vi "Splite Single-line Message.vi"(2 "Single-line Text":string) -> (6 "Operator":string, 7 "State":string, 9 "Args":string, 10 "Source/target":string)   [LabVIEW 2017, in "Communicable State Machine.lvlib"]
doc: "-- <b>Controls</b> --\n- <b>single-line text</b>:\n\n-- <b>Indicators</b> --\n- <b>operator</b>:\n- <b>state</b>:\n- <b>args</b>:\n- <b>source/target</b>:"
uses:
  Communicable State Machine.lvlib
  _Shared/CSM Shared.lvlib
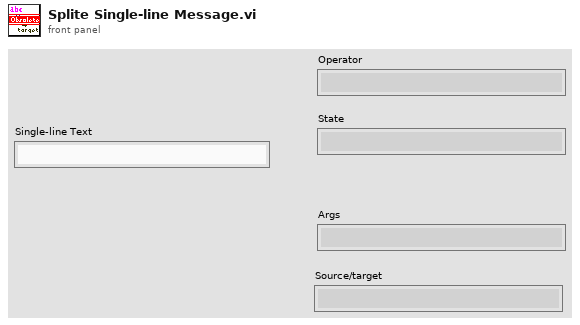
[diagram p1: front panel]
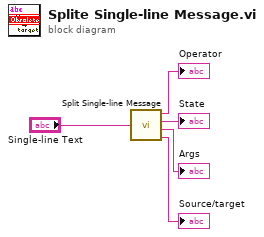
[diagram p0: block diagram]
diagram:
  n1 = call "Split Single-line Message.vi"("single-line text"="Single-line Text") -> ("operator"=→"Operator":string, "state"=→"State":string, "args"=→"Args":string, "source/target"=→"Source/target":string)  [unwired: 6 in]
